vi "Poly Refname to String.vi"   [LabVIEW 2014]
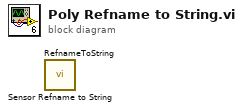
[diagram p0: block diagram]
diagram:
  n1 = call "Sensor Refname to String.vi"() -> ()  [unwired: 1 in, 1 out]
  n2 = call "RefnameToString.vi"() -> ()  [unwired: 1 in, 1 out]
